vi "ATF-Drive rotation State.vi"(6 "Drive_Enable":bool, 9 "Drive_Frequency":dbl, 10 "Drive_RPM":dbl, 11 "Drive_Status":bool) -> (3 "State":string)   [LabVIEW 2022 SP3]
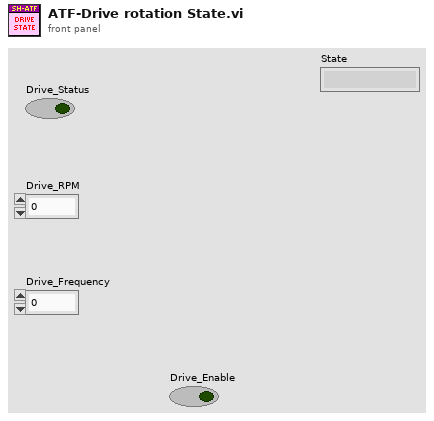
[diagram p1: front panel]
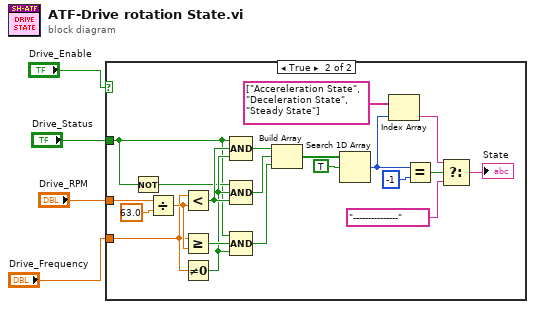
[diagram p0: block diagram]
diagram:
  n1 = case shown="True" "Drive_Enable" {
    tunnel: "Drive_RPM" -> [_ w19]
    tunnel: "Drive_Status" -> [_ w18]
    tunnel: "Drive_Frequency" -> [_ w17]
    frame False {
    }
    frame True {
      n2 = Not(x=w18) -> (.not. x?=w22:bool)
      n3 = Divide(x=w19, y=63.0 ("x")) -> (x/y=w20:dbl)
      n4 = Less?(x=w17, y=w20) -> (x < y?=w24:bool)
      n5 = Greater Or Equal?(x=w17, y=w20) -> (x >= y?=w25:bool)
      n6 = Not Equal To 0?(x=w17) -> (x != 0?=w23:bool)
      n7 = Compound Arithmetic op=AND(w18, w24, w23) -> (w15:bool)
      n8 = Compound Arithmetic op=AND(w22, w23, w24) -> (w14:bool)
      n9 = Compound Arithmetic op=AND(w18, w25, w23) -> (w13:bool)
      n10 = Build Array(w15, w14, w13) -> (w12:bool[])
      n11 = Search 1D Array(1D array=w12, element=TRUE) -> (index of element=w8:i32)  [unwired: 1 in]
      n12 = Index Array(array=string[] ["Accereleration State", "Deceleration State", "Steady State"], index=w8) -> (element=w9:string)
      n13 = Equal?(x=w8, y=-1) -> (x = y?=w6:bool)
      n14 = Select(t=w9, s=w6, f="---------------") -> (s? t:f=→"State":string)
    }
  }
